vi "[BLE Test] ble_read_write_characteristics.vi"() -> ()   [LabVIEW 2015]
uses:
  Lib_Bled112 toolkit/type_def/connection_status_bundle.ctl
  Lib_Bled112 toolkit/type_def/address_type.ctl
  Lib_Bled112 toolkit/type_def/message_type.ctl
  Lib_Bled112 toolkit/type_def/message_class.ctl
  Lib_Bled112 toolkit/ble_functions/ble_write_by_handle_uint8array.vi
panel:
  out "Rx Packet Structure":T1={"Message Type (Response)"=128, "Payload length"=0, "Command Class (System)"=1, "Message ID"=0, "Connection handle"=0, "Attribute handle"=0, "Attribute type"=1, "Attribute value (data)"=[]} {"Attribute type" format="%02x" items=["read", "notify", "indicate", "read_by_type", "read_blob", "indicate_rsp_req"]; "Attribute value (data)" format="%02x"; "Attribute handle" format="%04x"; "Connection handle" format="%02x"; "Message ID" format="%02x"; "Message Type (Response)" format="%02x" items=["Command / Response"=0, "Event"=128]; "Command Class (System)" format="%02x" items=["System", "Persistent Store", "Attribute database", "Connection", "Attribute client", "Security Manager", "Generic Access Profile", "Hardware"]}
  out "Packet Detect":bool=TRUE
  out "Disconnected":bool=TRUE
  out "Scan success?":bool
  out "BLED112 Dongle Info":string="Major: 1, Minor: 3, Patch: 2, Build: 122, LL ver: 3, Protocol ver: 1 and HW ver: 3  "
  out "그래프 타이머 값 1":u32=9582380
  out "CDC(PCAP02) Graph":waveform(sgl)[](graph)=[{"t0"=timestamp(3554331896.4574084 s since 1904-01-01), "dt"=0.03, "Y"=[1.0007696]}, {"t0"=timestamp(3554331896.4574084 s since 1904-01-01), "dt"=0.03, "Y"=[1.0004687]}]
  out "Working Time(H:M:S)":string="00:01:58"
  out "ms 타이머 값 2":u32=9464045
  in  "Device List":i32(listbox)=2
  out "Rx packet Interval graph":u32(graph)=30
  in  "Program Exit":bool=TRUE
  out "부분배열 2":u8[](array[numeric])=[253, 79, 255, 49, 255, 79, 255, 60, 255, 209, 65, 123, 0, 0, 0, 0, 0, 0, 0, 0] format="%x"
  out "Data-IMU":dbl=-3.014375 format="%.10f"
  out "Hex-IMU":i16=-689 format="%x"
  out "웨이브폼 차트-IMU":dbl(graph)=-3.014375
  in  "Index-IMU ch.":u8(slide)=1 min=1 max=6 step=1 scale=1.0..6.0
  out "Rx OK":bool=TRUE
  out "ms 타이머 값":u32=9582439
  out "Entire-Rx time(ms)":i32=30
  in  "Index-CDC ch.":u8(slide)=1 min=1 max=6 step=1 scale=1.0..6.0
  out "웨이브폼 차트 - CDC":sgl(graph)=1.0007696
  out "Hex-CDC":u32=2098766 format="%x"
  out "Data-CDC":dbl=1.0007696151733398 format="%.10f"
  out "부분배열":u8[](array[numeric])=[32, 6, 78, 32, 3, 215, 32, 6, 110, 32, 71, 249, 32, 115, 92, 32, 30, 38, 1, 0] format="%x"
  in  "Tx 문자열":string="\nBLED112 Test\n"
  in  "Tx Send":bool
  out "Rx Cnt":i32=3775
  in  "Rx Stop":bool=TRUE
  out "Rx 문자열 1":string
  out "Connected":bool
  out "Device Name":string
  out "Address Type":enum16{"Public", "Random"}(ring)=enum."Random"
  out "Handle table":string[][](array[string])
  out "Connection Status":T4 {"Address Type" items=["Public", "Random"]}
  out "Scanning":bool
  in  "Device Connect":bool=TRUE
  out "MAC Address":string="D9:2F:10:92:34:F2"
  in  "COM Bluegiga in":refnum<visa-resource-name>="COM8"
  # "GEN4 1st PP - BLE(Bluetooth Low Energy) Test"
  # "CDC Data"
  # "SCAN"
  # "DEVICES FOUND"
  # "CONNECT"
  # "Introduce the MAC Address and Address Type of the device you want to connect and click in the CONTINUE button"
  # "IMU Data"
  # "Service 0x1800\nCharacteristic 0x2A00\nDevice Name"
  # "READING DEVICE NAME"
  # "Read"
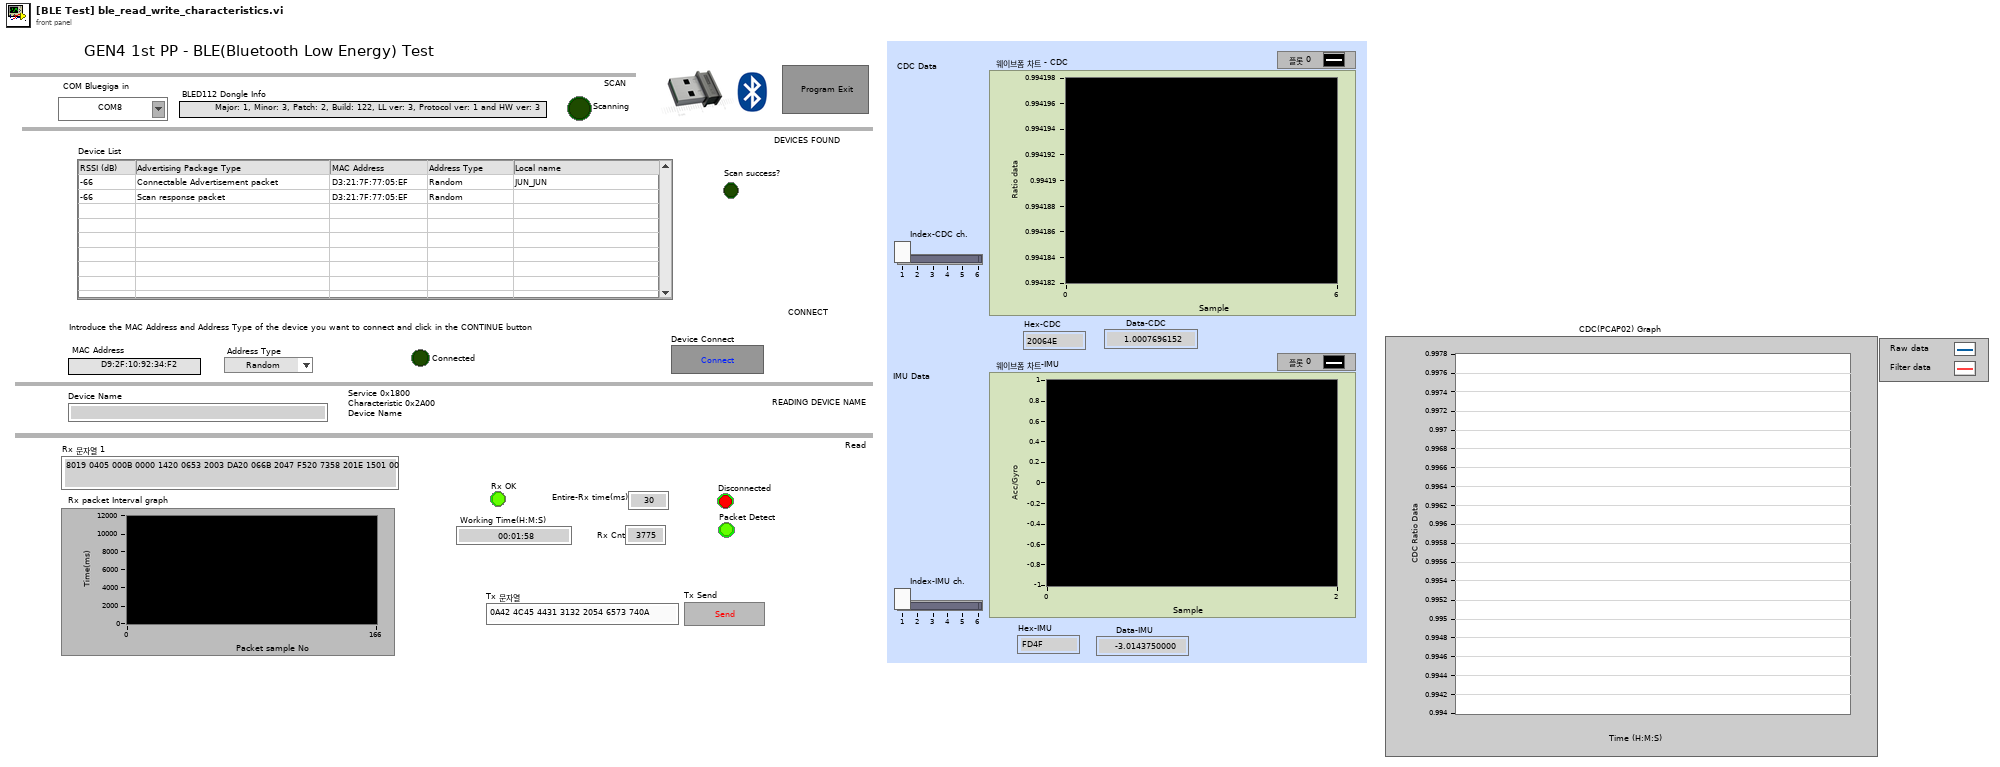
[diagram p1: front panel]
types:
  T1 = typedef "컨트롤-BLED Rx (EVENT-Attribute Client).ctl" = cluster{"Message Type (Response)":T2, "Payload length":u8, "Command Class (System)":T3, "Message ID":u8, "Connection handle":u8, "Attribute handle":u16, "Attribute type":T3, "Attribute value (data)":u8[]}
  T2 = typedef "message_type.ctl" = u8
  T3 = typedef "message_class.ctl" = u8
  T4 = typedef "connection_status_bundle.ctl" = cluster{"MAC Address":string, "cnx handle":u8, "cnx flags":u8, "Address Type":T5, "Connection Interval (ms)":u16, "Timeout(ms)":u16, "Latency":u16, "bonding handle":u8}
  T5 = typedef "address_type.ctl" = u8
  T6 = typedef "컨트롤-BLED Rx (EVENT-Connection status).ctl" = cluster{"Message Type (Response)":T2, "Payload length":u8, "Command Class (System)":T3, "Message ID":u8, "Connection handle":u8, "flags":u8, "Bluetooth address":u8[], "address type":T3, "conn_interval(ms)":dbl, "timeout(ms)":dbl, "latency":u16, "bonding(0xFF)":u8}
  T7 = typedef "컨트롤-BLED Rx (EVENT-Disconnected).ctl" = cluster{"Message Type (Response)":T2, "Payload length":u8, "Command Class (Connection)":T3, "Message ID":u8, "connection":u8, "reason":u16}
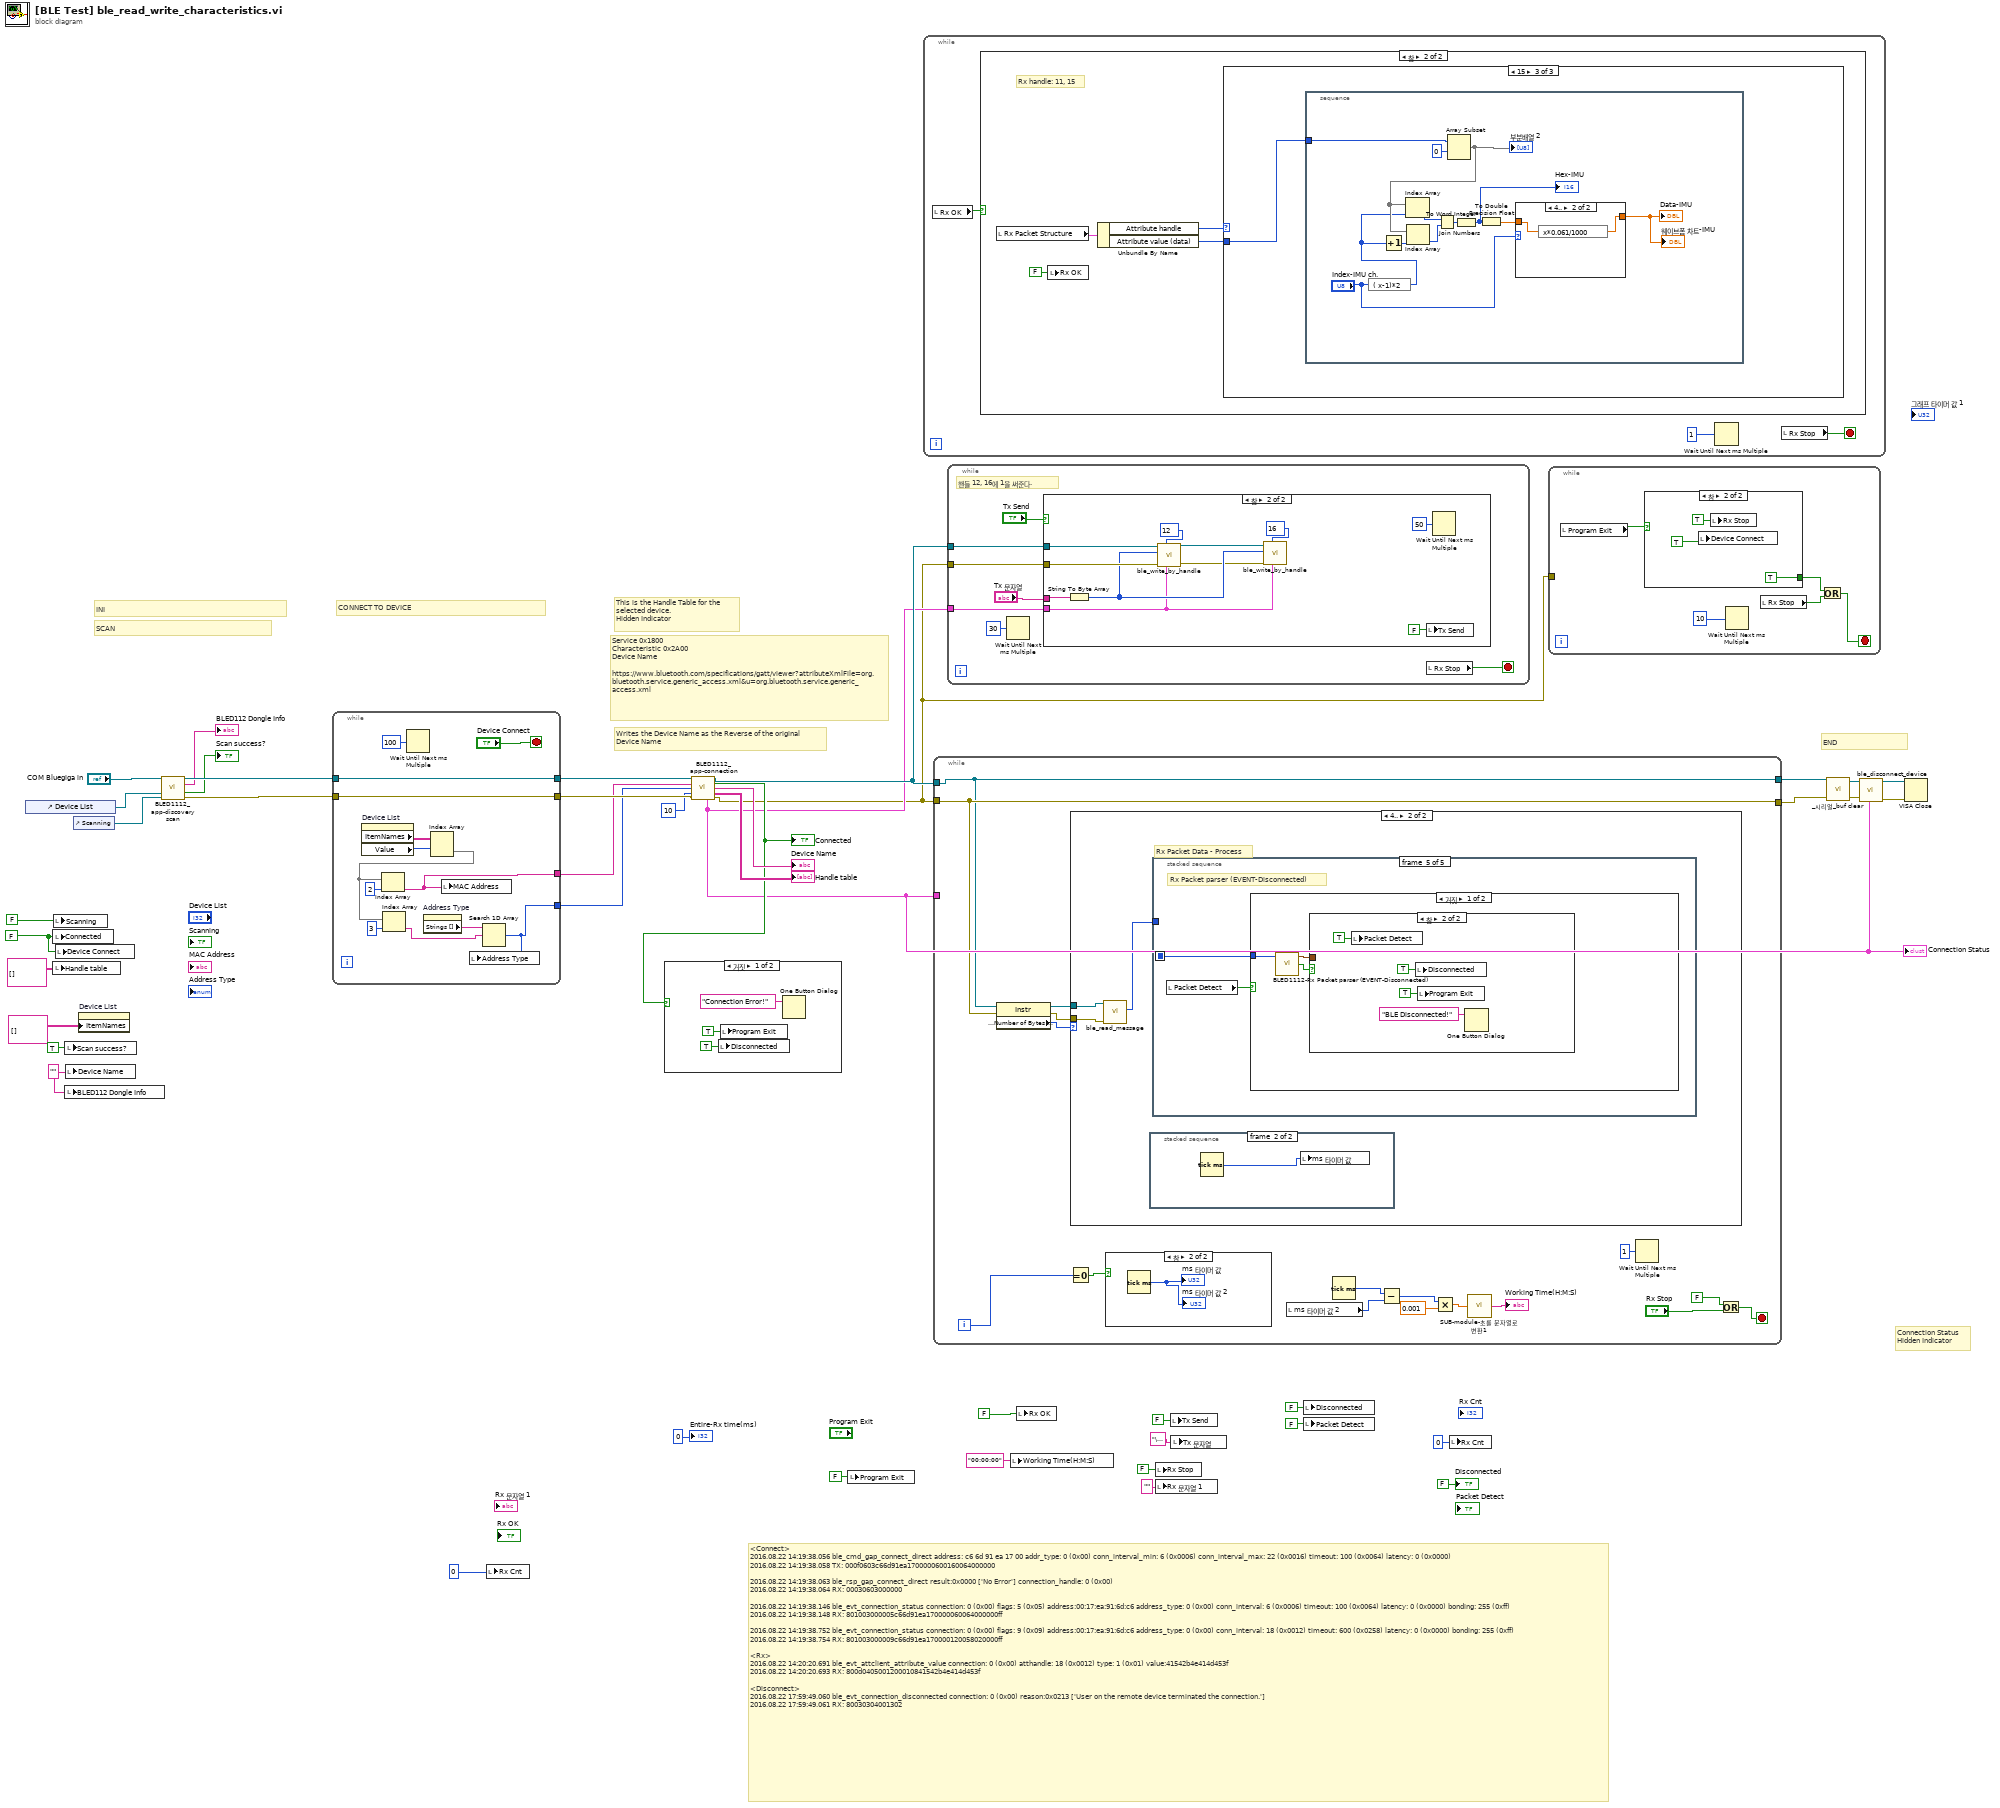
[diagram p0: block diagram]
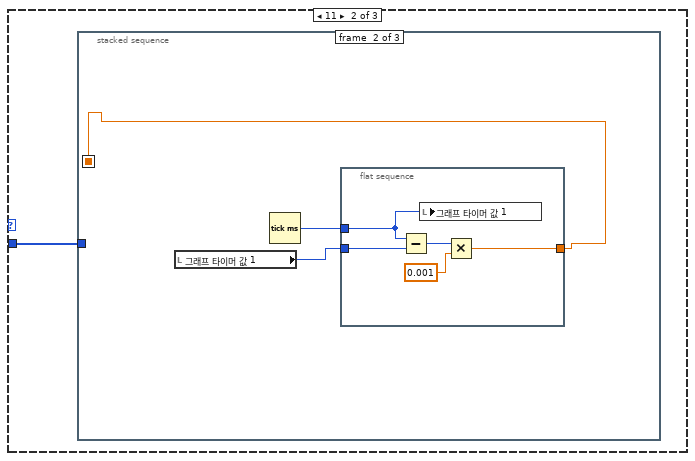
[diagram p7: hidden frame]
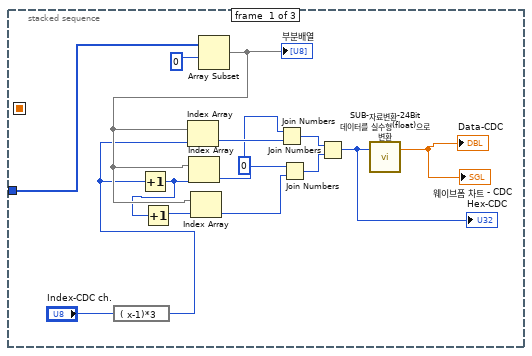
[diagram p8: hidden frame]
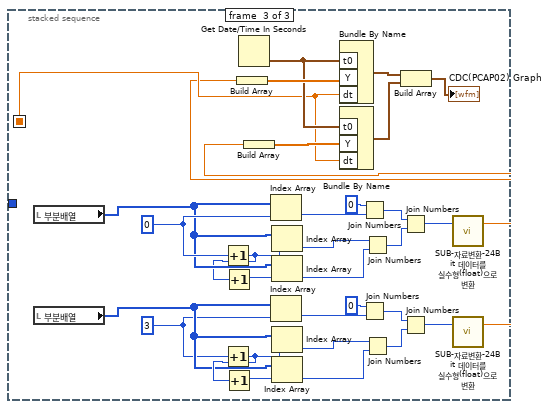
[diagram p9: hidden frame]
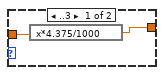
[diagram p10: hidden frame]
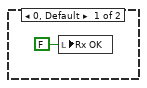
[diagram p11: hidden frame]
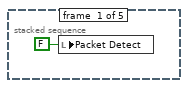
[diagram p12: hidden frame]
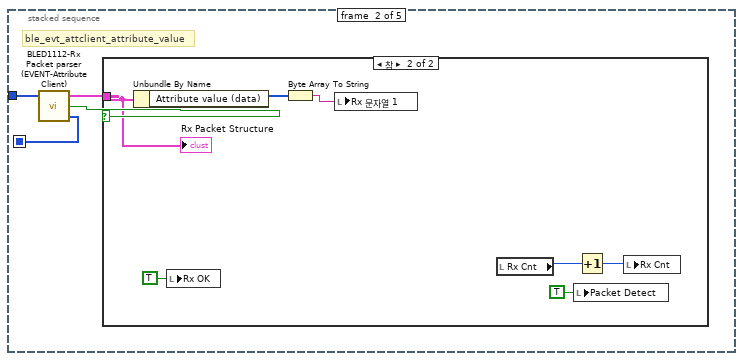
[diagram p13: hidden frame]
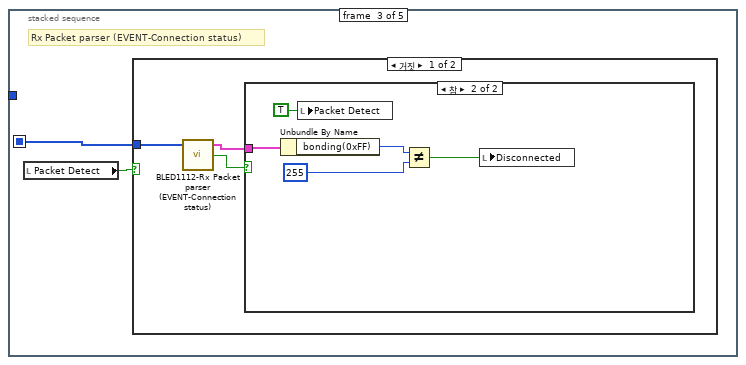
[diagram p15: hidden frame]
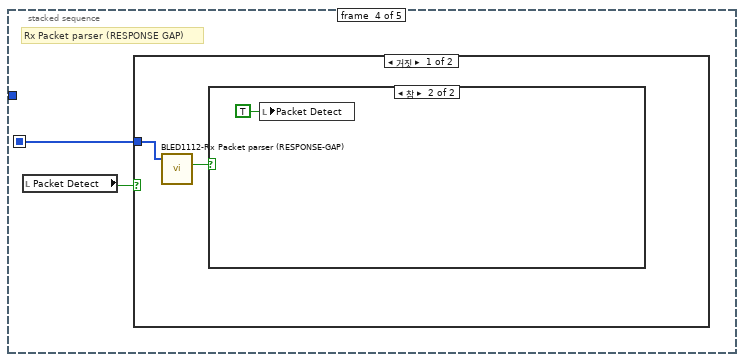
[diagram p18: hidden frame]
diagram:
  w19 = "" ("Device Name")
  w40 = FALSE ("Connected")
  # "<Connect>\n2016.08.22 14:19:38.056 ble_cmd_gap_connect_direct address: c6 6d 91 ea 17 00 addr_type: 0 (0x00) conn_interval_min: 6 (0x0006) conn_interval_max: 22 (0x0016) timeout: 100 (0x0064) latency: 0 (0x0000)\n2016.08.22 14:19:38.058 TX: 000f0603c66d91ea1700000600160064000000\n\n2016.08.22 14:19:38.063 ble_rsp_gap_connect_direct result:0x0000 ['No Error'] connection_handle: 0 (0x00)\n2016.08.22 14:19:38.064 RX: 00030603000000\n\n2016.08.22 14:19:38.146 ble_evt_connection_status connection: 0 (0x00) flags: 5 (0x05) address:00:17:ea:91:6d:c6 address_type: 0 (0x00) conn_interval: 6 (0x0006) timeout: 100 (0x0064) latency: 0 (0x0000) bonding: 255 (0xff)\n2016.08.22 14:19:38.148 RX: 801003000005c66d91ea170000060064000000ff\n\n2016.08.22 14:19:38.752 ble_evt_connection_status connection: 0 (0x00) flags: 9 (0x09) address:00:17:ea:91:6d:c6 address_type: 0 (0x00) conn_interval: 18 (0x0012) timeout: 600 (0x0258) latency: 0 (0x0000) bonding: 255 (0xff)\n2016.08.22 14:19:38.754 RX: 801003000009c66d91ea170000120058020000ff\n\n<Rx>\n2016.08.22 14:20:20.691 ble_evt_attclient_attribute_value connection: 0 (0x00) atthandle: 18 (0x0012) type: 1 (0x01) value:41542b4e414d453f\n2016.08.22 14:20:20.693 RX: 800d0405001200010841542b4e414d453f\n\n<Disconnect>\n2016.08.22 17:59:49.060 ble_evt_connection_disconnected connection: 0 (0x00) reason:0x0213 ['User on the remote device terminated the connection.']\n2016.08.22 17:59:49.061 RX: 80030304001302"
  # "Writes the Device Name as the Reverse of the original\nDevice Name"
  # "Service 0x1800\nCharacteristic 0x2A00\nDevice Name\n\nhttps://www.bluetooth.com/specifications/gatt/viewer?attributeXmlFile=org.bluetooth.service.generic_access.xml&u=org.bluetooth.service.generic_access.xml"
  # "This is the Handle Table for the\nselected device. \nHidden Indicator"
  # "Connection Status\nHidden Indicator"
  # "CONNECT TO DEVICE"
  # "SCAN"
  # "END"
  # "INI"
  n1 = control-ref of="Device List"() -> (w23:refnum<vi>)
  n2 = local write "Connected"(w40) -> ()
  n3 = local write "Handle table"(string[][] [] ("Handle table")) -> ()
  n4 = local write "Scanning"(FALSE ("Scanning")) -> ()
  n5 = local write "Device Connect"(w40) -> ()
  n6 = local write "Scan success?"(TRUE ("Scan success?")) -> ()
  n7 = local write "BLED112 Dongle Info"(w19) -> ()
  n8 = local write "Device Name"(w19) -> ()
  n9 = control-ref of="Scanning"() -> (w22:refnum<vi>)
  n10 = property on="Device List" class="MCListbox (엄격한)"("ItemNames"=string[][] [] ("Devices")) -> ()  [unwired: 2 in, 2 out]
  n11 = call "BLED1112_app-discovery scan.vi"("COM in"="COM Bluegiga in", "Device List"=w23, "LED ref"=w22) -> ("COM out"=w21:refnum<visa-resource-name>, "BLED112 Dongle Info"=→"BLED112 Dongle Info":string, "Scan success?"=→"Scan success?":bool, "error out"=w18:errorcluster)  [unwired: 8 in, 1 out]
  n12 = while {
    tunnel: w18 -> [w45]
    tunnel: [w55] -> w11
    tunnel: w21 -> [w55]
    tunnel: [w45] -> w10
    tunnel: [w51] -> w9
    tunnel: [w46] -> w8
    stop <- "Device Connect" stop-if-true
    n13 = property on="Device List" class="MCListbox (엄격한)"() -> ("ItemNames"=w54:string[][], "Value"=w53:i32)  [unwired: 2 in, 2 out]
    n14 = Wait Until Next ms Multiple(millisecond multiple=u32 100 ("ms 배수")) -> ()  [unwired: 1 out]
    n15 = property on="Address Type" class="Enum (엄격한)"() -> ("Strings []"=w48:string[])  [unwired: 2 in, 2 out]
    n16 = Index Array(array=w54, index (row)=w53) -> (element=w49:string[])  [unwired: 1 in]
    n17 = Index Array(array=w49, index=2 ("인덱스")) -> (element=w51:string)
    n18 = Index Array(array=w49, index=3 ("인덱스")) -> (element=w47:string)
    n19 = local write "MAC Address"(w51) -> ()
    n20 = Search 1D Array(1D array=w48, element=w47) -> (index of element=w46:i32)  [unwired: 1 in]
    n21 = local write "Address Type"(w46) -> ()
  }
  n22 = local write "Rx Cnt"(u32 0 ("CDC-Rx time(ms)")) -> ()
  n23 = call "BLED1112_app-connection.vi"("COM Bluegiga in"=w11, "MAC Address"=w9, "Address Type"=w8, "Conn Try no"=10, "error in"=w10) -> ("COM out"=w7:refnum<visa-resource-name>, "Connection Ok"=w3:bool, "Device Name"=→"Device Name":string, "Handle table"=→"Handle table":string[][], "Connection Status"=w2:T4, "에러 출력"=w1:errorcluster)  [unwired: 5 in]
  "Connection Status" <- w2
  "Connected" <- w3
  n24 = case shown="거짓" w3 {
    frame False {
      n25 = local write "Disconnected"(TRUE ("Disconnected")) -> ()
      n26 = local write "Program Exit"(TRUE ("정지")) -> ()
      n27 = One Button Dialog(message="Connection Error!" ("메시지")) -> ()  [unwired: 1 in, 1 out]
    }
    frame True {
    }
  }
  n28 = local write "Program Exit"(FALSE ("정지")) -> ()
  n29 = while {
    stop <- w62 stop-if-true
    n30 = local read "Rx OK"() -> (w60:bool)
    n31 = case shown="참" w60 {
      frame False {
      }
      frame True {
        # "Rx handle: 11, 15"
        n32 = local read "Rx Packet Structure"() -> (w66:T1)
        n33 = local write "Rx OK"(FALSE ("Rx OK")) -> ()
        n34 = Unbundle By Name(w66) -> ("Attribute handle"=w65:u16, "Attribute value (data)"=w63:u8[])
        n35 = case shown="15" w65 {
          tunnel: w63 -> [_ w67 w122]
          frame 0, Default {
          }
          frame 11 {
            n36 = stacked-sequence {
              seq-local: [_ w83 _] -> [_ _ w115]
              tunnel: w67 -> [w68 _ _]
              frame #0 {
                n37 = expression code="( x-1)*3"("Index-CDC ch.") -> (w71:u8)
                n38 = Increment(x=w71) -> (x+1=w70:u8)
                n39 = Increment(x=w70) -> (x+1=w69:u8)
                n40 = Array Subset(array=w68, index=0 ("인덱스")) -> (w81:u8[])  [unwired: 1 in]
                "부분배열" <- w81
                n41 = Index Array(array=w81, index=w71) -> (element=w78:u8)
                n42 = Index Array(array=w81, index=w70) -> (element=w79:u8)
                n43 = Index Array(array=w81, index=w69) -> (element=w80:u8)
                n44 = Join Numbers(hi=u8 0 ("인덱스"), lo=w78) -> ((hi.lo)=w75:u16)
                n45 = Join Numbers(hi=w79, lo=w80) -> ((hi.lo)=w76:u16)
                n46 = Join Numbers(hi=w75, lo=w76) -> ((hi.lo)=w74:u32)
                "Hex-CDC" <- w74
                n47 = call "SUB-자료변환-24Bit 데이터를 실수형(float)으로 변환.vi"("U32"=w74) -> ("FP32"=→"Data-CDC" →"웨이브폼 차트 - CDC":sgl)  [unwired: 2 in]
              }
              frame #1 {
                n48 = local read "그래프 타이머 값 1"() -> (w85:u32)
                n49 = Tick Count (ms)() -> (millisecond timer value=w84:u32)
                n50 = flat-sequence {
                  tunnel: w84 -> [w90]
                  tunnel: w85 -> [w87]
                  tunnel: [w86] -> w83
                  frame #0 {
                    n51 = Subtract(x=w90, y=w87) -> (x-y=w88:u32)
                    n52 = local write "그래프 타이머 값 1"(w90) -> ()
                    n53 = Multiply(x=w88, y=0.001 ("dt")) -> (x*y=w86:dbl)
                  }
                }
              }
              frame #2 {
                w93 = u8 3 ("인덱스")
                w114 = u8 0 ("인덱스")
                n54 = local read "부분배열"() -> (w113:u8[])
                n55 = local read "부분배열"() -> (w94:u8[])
                n56 = Increment(x=w114) -> (x+1=w105:u8)
                n57 = Increment(x=w93) -> (x+1=w102:u8)
                n58 = Increment(x=w105) -> (x+1=w104:u8)
                n59 = Increment(x=w102) -> (x+1=w103:u8)
                n60 = Get Date/Time In Seconds() -> (seconds since 1Jan1904=w119:timestamp)
                n61 = Index Array(array=w113, index=w114) -> (element=w110:u8)
                n62 = Index Array(array=w94, index=w93) -> (element=w97:u8)
                n63 = Index Array(array=w113, index=w105) -> (element=w111:u8)
                n64 = Index Array(array=w113, index=w104) -> (element=w112:u8)
                n65 = Index Array(array=w94, index=w102) -> (element=w96:u8)
                n66 = Index Array(array=w94, index=w103) -> (element=w95:u8)
                n67 = Join Numbers(hi=u8 0 ("인덱스"), lo=w110) -> ((hi.lo)=w107:u16)
                n68 = Join Numbers(hi=u8 0 ("인덱스"), lo=w97) -> ((hi.lo)=w100:u16)
                n69 = Join Numbers(hi=w111, lo=w112) -> ((hi.lo)=w108:u16)
                n70 = Join Numbers(hi=w96, lo=w95) -> ((hi.lo)=w99:u16)
                n71 = Join Numbers(hi=w107, lo=w108) -> ((hi.lo)=w106:u32)
                n72 = Join Numbers(hi=w100, lo=w99) -> ((hi.lo)=w101:u32)
                n73 = call "SUB-자료변환-24Bit 데이터를 실수형(float)으로 변환.vi"("U32"=w106) -> ("FP32"=w92:sgl)  [unwired: 2 in]
                n74 = Build Array(w92) -> (w120:sgl[])
                n75 = Bundle By Name("t0"=w119, "Y"=w120, "dt"=w115) -> (w116:waveform(sgl))  [unwired: 1 in]
                n76 = call "SUB-자료변환-24Bit 데이터를 실수형(float)으로 변환.vi"("U32"=w101) -> ("FP32"=w91:sgl)  [unwired: 2 in]
                n77 = Build Array(w91) -> (w121:sgl[])
                n78 = Bundle By Name("t0"=w119, "Y"=w121, "dt"=w115) -> (w117:waveform(sgl))  [unwired: 1 in]
                n79 = Build Array(w116, w117) -> (→"CDC(PCAP02) Graph":waveform(sgl)[])
              }
            }
          }
          frame 15 {
            n80 = stacked-sequence {
              tunnel: w122 -> [w123]
              frame #0 {
                n81 = expression code="( x-1)*2"("Index-IMU ch.") -> (w127:u8)
                n82 = Increment(x=w127) -> (x+1=w126:u8)
                n83 = Array Subset(array=w123, index=0 ("인덱스")) -> (w133:u8[])  [unwired: 1 in]
                "부분배열 2" <- w133
                n84 = Index Array(array=w133, index=w127) -> (element=w132:u8)
                n85 = Index Array(array=w133, index=w126) -> (element=w131:u8)
                n86 = Join Numbers(hi=w132, lo=w131) -> ((hi.lo)=w129:u16)
                n87 = To Word Integer(number=w129) -> (16bit integer=w125:i16)
                "Hex-IMU" <- w125
                n88 = To Double Precision Float(number=w125) -> (double precision float=w128:dbl)
                n89 = case shown="4.." "Index-IMU ch." {
                  tunnel: [w136 w137] -> w130
                  tunnel: w128 -> [w135 w138]
                  frame ..3 {
                    n90 = expression code="x*4.375/1000"(w135) -> (w136:dbl)
                  }
                  frame 4.. {
                    n91 = expression code="x*0.061/1000"(w138) -> (w137:dbl)
                  }
                }
                "Data-IMU" <- w130
                "웨이브폼 차트-IMU" <- w130
              }
            }
          }
        }
      }
    }
    n92 = Wait Until Next ms Multiple(millisecond multiple=u32 1 ("ms 배수")) -> ()  [unwired: 1 out]
    n93 = local read "Rx Stop"() -> (w62:bool)
  }
  n94 = while {
    tunnel: w7 -> [w142]
    tunnel: w1 -> [w143]
    tunnel: w2 -> [_]
    tunnel: [w142] -> w38
    tunnel: [w143] -> w37
    i -> [w153]
    stop <- w154 stop-if-true
    n95 = property class="Instr"(reference=w142, error in=w143) -> (reference out=w140:refnum<visa-resource-name>, error out=w139:errorcluster, "Serial Settings:Number of Bytes at Serial Port"=w141:u32)
    n96 = Equal To 0?(x=w153) -> (x = 0?=w152:bool)
    n97 = case shown="4.." w141 {
      tunnel: w140 -> [_ w159]
      tunnel: w139 -> [_ w158]
      frame 0, Default {
        n98 = local write "Rx OK"(FALSE ("Rx OK")) -> ()
      }
      frame 4.. {
        # "Rx Packet Data - Process"
        n99 = call "ble_read_message.vi"("error in (no error)"=w158, "COM Bluegiga in"=w159) -> ("message package"=w157:u8[])  [unwired: 7 in, 2 out]
        n100 = stacked-sequence {
          frame #0 {
            n101 = local read "ms 타이머 값"() -> (w198:u32)
            n102 = Tick Count (ms)() -> (millisecond timer value=w197:u32)
            n103 = Subtract(x=w197, y=w198) -> (x-y=w196:u32)
            "Rx packet Interval graph" <- w196
            n104 = local write "Entire-Rx time(ms)"(w196) -> ()
          }
          frame #1 {
            n105 = Tick Count (ms)() -> (millisecond timer value=w199:u32)
            n106 = local write "ms 타이머 값"(w199) -> ()
          }
        }
        n107 = stacked-sequence {
          seq-local: [_ w162 _ _ _] -> [_ _ w173 w183 w188]
          tunnel: w157 -> [_ w163 _ _ _]
          frame #0 {
            n108 = local write "Packet Detect"(FALSE ("Packet Detect")) -> ()
          }
          frame #1 {
            # "ble_evt_attclient_attribute_value"
            n109 = call "BLED1112-Rx Packet parser (EVENT-Attribute Client).vi"("message package"=w163) -> ("message out"=w162:u8[], "Packet OK"=w161:bool, "Data Structure"=w164:T1)  [unwired: 2 in]
            n110 = case shown="참" w161 {
              tunnel: w164 -> [_ w169]
              frame False {
              }
              frame True {
                n111 = Unbundle By Name(w169) -> ("Attribute value (data)"=w167:u8[])
                n112 = local write "Rx OK"(TRUE ("Rx OK")) -> ()
                n113 = Byte Array To String(unsigned byte array=w167) -> (string=w168:string)
                n114 = local write "Rx 문자열 1"(w168) -> ()
                n115 = local read "Rx Cnt"() -> (w170:i32)
                n116 = local write "Packet Detect"(TRUE ("Packet Detect")) -> ()
                n117 = Increment(x=w170) -> (x+1=w171:i32)
                n118 = local write "Rx Cnt"(w171) -> ()
                "Rx Packet Structure" <- w169
              }
            }
          }
          frame #2 {
            # "Rx Packet parser (EVENT-Connection status)"
            n119 = local read "Packet Detect"() -> (w172:bool)
            n120 = case shown="거짓" w172 {
              tunnel: w173 -> [w176 _]
              frame False {
                n121 = call "BLED1112-Rx Packet parser (EVENT-Connection status).vi"("message package"=w176) -> ("Packet OK"=w175:bool, "Data Structure"=w174:T6)  [unwired: 2 in, 1 out]
                n122 = case shown="참" w175 {
                  tunnel: w174 -> [_ w181]
                  frame False {
                  }
                  frame True {
                    n123 = Unbundle By Name(w181) -> ("bonding(0xFF)"=w180:u8)
                    n124 = local write "Packet Detect"(TRUE ("Packet Detect")) -> ()
                    n125 = Not Equal?(x=w180, y=255 ("Rx Cnt")) -> (x != y?=w178:bool)
                    n126 = local write "Disconnected"(w178) -> ()
                  }
                }
              }
              frame True {
              }
            }
          }
          frame #3 {
            # "Rx Packet parser (RESPONSE GAP)"
            n127 = local read "Packet Detect"() -> (w182:bool)
            n128 = case shown="거짓" w182 {
              tunnel: w183 -> [w185 _]
              frame False {
                n129 = call "BLED1112-Rx Packet parser (RESPONSE-GAP).vi"("message package"=w185) -> ("Packet OK"=w184:bool)  [unwired: 2 in, 2 out]
                n130 = case shown="참" w184 {
                  frame False {
                  }
                  frame True {
                    n131 = local write "Packet Detect"(TRUE ("Packet Detect")) -> ()
                  }
                }
              }
              frame True {
              }
            }
          }
          frame #4 {
            # "Rx Packet parser (EVENT-Disconnected)"
            n132 = local read "Packet Detect"() -> (w187:bool)
            n133 = case shown="거짓" w187 {
              tunnel: w188 -> [w190 _]
              frame False {
                n134 = call "BLED1112-Rx Packet parser (EVENT-Disconnected).vi"("message package"=w190) -> ("Packet OK"=w191:bool, "Data Structure"=w189:T7)  [unwired: 2 in, 1 out]
                n135 = case shown="참" w191 {
                  tunnel: w189 -> [_ _]
                  frame False {
                  }
                  frame True {
                    n136 = local write "Packet Detect"(TRUE ("Packet Detect")) -> ()
                    n137 = local write "Disconnected"(TRUE ("Disconnected")) -> ()
                    n138 = local write "Program Exit"(TRUE ("정지")) -> ()
                    n139 = One Button Dialog(message="BLE Disconnected!" ("메시지")) -> ()  [unwired: 1 in, 1 out]
                  }
                }
              }
              frame True {
              }
            }
          }
        }
      }
    }
    n140 = case shown="참" w152 {
      frame False {
      }
      frame True {
        n141 = Tick Count (ms)() -> (millisecond timer value=→"ms 타이머 값" →"ms 타이머 값 2":u32)
      }
    }
    n142 = local read "ms 타이머 값 2"() -> (w150:u32)
    n143 = Tick Count (ms)() -> (millisecond timer value=w151:u32)
    n144 = Subtract(x=w151, y=w150) -> (x-y=w147:u32)
    n145 = Multiply(x=w147, y=0.001) -> (x*y=w149:dbl)
    n146 = call "SUB-module-초를 문자열로 변환1.vi"("입력-초단위"=w149) -> ("시:분:초"=→"Working Time(H:M:S)":string)
    n147 = Wait Until Next ms Multiple(millisecond multiple=u32 1 ("ms 배수")) -> ()  [unwired: 1 out]
    n148 = Or(x=FALSE, y="Rx Stop") -> (x .or. y?=w154:bool)
  }
  n149 = while {
    tunnel: w7 -> [w204]
    tunnel: w1 -> [w203]
    tunnel: w2 -> [w201]
    stop <- w205 stop-if-true
    # "핸들 12, 16에 1을 써준다."
    n150 = Wait Until Next ms Multiple(millisecond multiple=u32 30 ("ms 배수")) -> ()  [unwired: 1 out]
    n151 = case shown="참" "Tx Send" {
      tunnel: w204 -> [_ w218]
      tunnel: w203 -> [_ w217]
      tunnel: "Tx 문자열" -> [_ w212]
      tunnel: w201 -> [_ w208]
      frame False {
      }
      frame True {
        n152 = String To Byte Array(string=w212) -> (unsigned byte array=w211:u8[])
        n153 = call-poly "ble_write_by_handle.vi"("Connection Status"=w208, "Handle"=u16 12, "error in (no error)"=w217, "data (uint8array)"=w211, "COM Bluegiga in"=w218) -> ("error out"=w209:errorcluster, "COM Bluegiga out"=w210:refnum<visa-resource-name>)  [unwired: 5 in]
        n154 = call-poly "ble_write_by_handle.vi"("Connection Status"=w208, "Handle"=u16 16, "error in (no error)"=w209, "data (uint8array)"=w211, "COM Bluegiga in"=w210) -> ()  [unwired: 5 in, 2 out]
        n155 = local write "Tx Send"(FALSE ("Tx Send")) -> ()
        n156 = Wait Until Next ms Multiple(millisecond multiple=u32 50 ("ms 배수")) -> ()  [unwired: 1 out]
      }
    }
    n157 = local read "Rx Stop"() -> (w205:bool)
  }
  n158 = local write "Working Time(H:M:S)"("00:00:00" ("Working Time(H:M:S)")) -> ()
  n159 = local write "Rx OK"(FALSE ("success?")) -> ()
  n160 = local write "Rx Stop"(FALSE ("Rx 정지")) -> ()
  n161 = local write "Rx 문자열 1"("" ("Rx 문자열")) -> ()
  n162 = local write "Tx Send"(FALSE ("Tx Send")) -> ()
  n163 = local write "Tx 문자열"("\u0001" ("Tx 문자열")) -> ()
  n164 = local write "Disconnected"(FALSE ("Disconnected")) -> ()
  n165 = local write "Packet Detect"(FALSE ("Packet Detect")) -> ()
  n166 = local write "Rx Cnt"(0 ("Rx Cnt")) -> ()
  n167 = while {
    tunnel: w1 -> [_]
    stop <- w219 stop-if-true
    n168 = local read "Program Exit"() -> (w223:bool)
    n169 = case shown="참" w223 {
      tunnel: [_ TRUE] -> w220
      frame False {
      }
      frame True {
        n170 = local write "Device Connect"(TRUE ("Continue")) -> ()
        n171 = local write "Rx Stop"(TRUE ("Rx 정지")) -> ()
      }
    }
    n172 = Wait Until Next ms Multiple(millisecond multiple=u32 10 ("ms 배수")) -> ()  [unwired: 1 out]
    n173 = local read "Rx Stop"() -> (w221:bool)
    n174 = Or(x=w220, y=w221) -> (x .or. y?=w219:bool)
  }
  n175 = call "_시리얼_buf clear.vi"("에러 출력 2"=w37, "시리얼 포트"=w38) -> ("에러 출력"=w26:errorcluster, "시리얼 포트 2"=w25:refnum<visa-resource-name>)  [unwired: 2 in]
  n176 = call "ble_disconnect_device.vi"("Connection Status"=w2, "error in (no error)"=w26, "COM Bluegiga in"=w25) -> ("error out"=w42:errorcluster, "COM Bluegiga out"=w43:refnum<visa-resource-name>)  [unwired: 7 in]
  n177 = VISA Close(VISA resource name=w43, error in (no error)=w42) -> ()  [unwired: 1 out]
  "Entire-Rx time(ms)" <- 0 ("수신 주기(ms)")
  "Disconnected" <- FALSE ("packer Parser")
